vi "Module Top Level.vi"(8 "error in":errorcluster) -> (0 "error out":errorcluster)   [LabVIEW 2018, in "Fuel Farm.lvlib"]
doc: "This is the top level VI for this module. It uses a queue for communications and is stopped user a user event. The general architecture is similar to a simple queued message handler.\n\nThe VIs associated with this module are organized in a LabVIEW Library."
uses:
  Fuel Farm.lvlib
  Private Controls/UI 3 Data.ctl
  Top Level/Shared Controls/APU Setup File.ctl
  Testing UI 1/Private Controls/APU & ECU Controls.ctl
  Private Controls/Module Data.ctl
  Private Controls/Module Action.ctl
  Controller (Host)/Public Controls/APU Select.ctl
  <vilib>/event_ctls.llb/usereventprio.ctl
  Globals/Host Globals.vi
  Error Handler/Error Handler.lvlib
  Controller (Host)/Controller (Host).lvlib
  File IO/File IO.lvlib
  UDP Writer/PC UDP Writer.lvlib
  Testing UI 1/Testing UI 1.lvlib
panel:
  out "cRIO Status":bool
  in  "FuelSystem":bool caption="FUEL SYSTEM"
  in  "Pressure Regulator":dbl(slide)=4.0 min=4.0 max=20.0 step=0.1 scale=4.0..20.0 scale format="%_2g"
  out "01.00.9213.09":cluster{dbl, dbl, dbl, dbl}(slide)={0.0, 380.23952095808386, 305.38922155688624, 392.21556886227546} caption="Tamb" scale=0.0..200.0 scale format="%.2f F"
  out "01.00.9213.09":dbl(slide) caption="TFFT" scale=0.0..200.0
  out "C.36":dbl(slide) caption="Flow" scale=0.0..2000.0
  out "Fuel Pressure":dbl caption="PFI" format="%.2g"
  out "02.03.9227.03":dbl(slide)=100.0 caption="Level" scale=0.0..100.0
  out "UI 3 Data":T1
  out "STOP":bool
  # "Fuel Farm"
  # "Decrease"
  # "Increase"
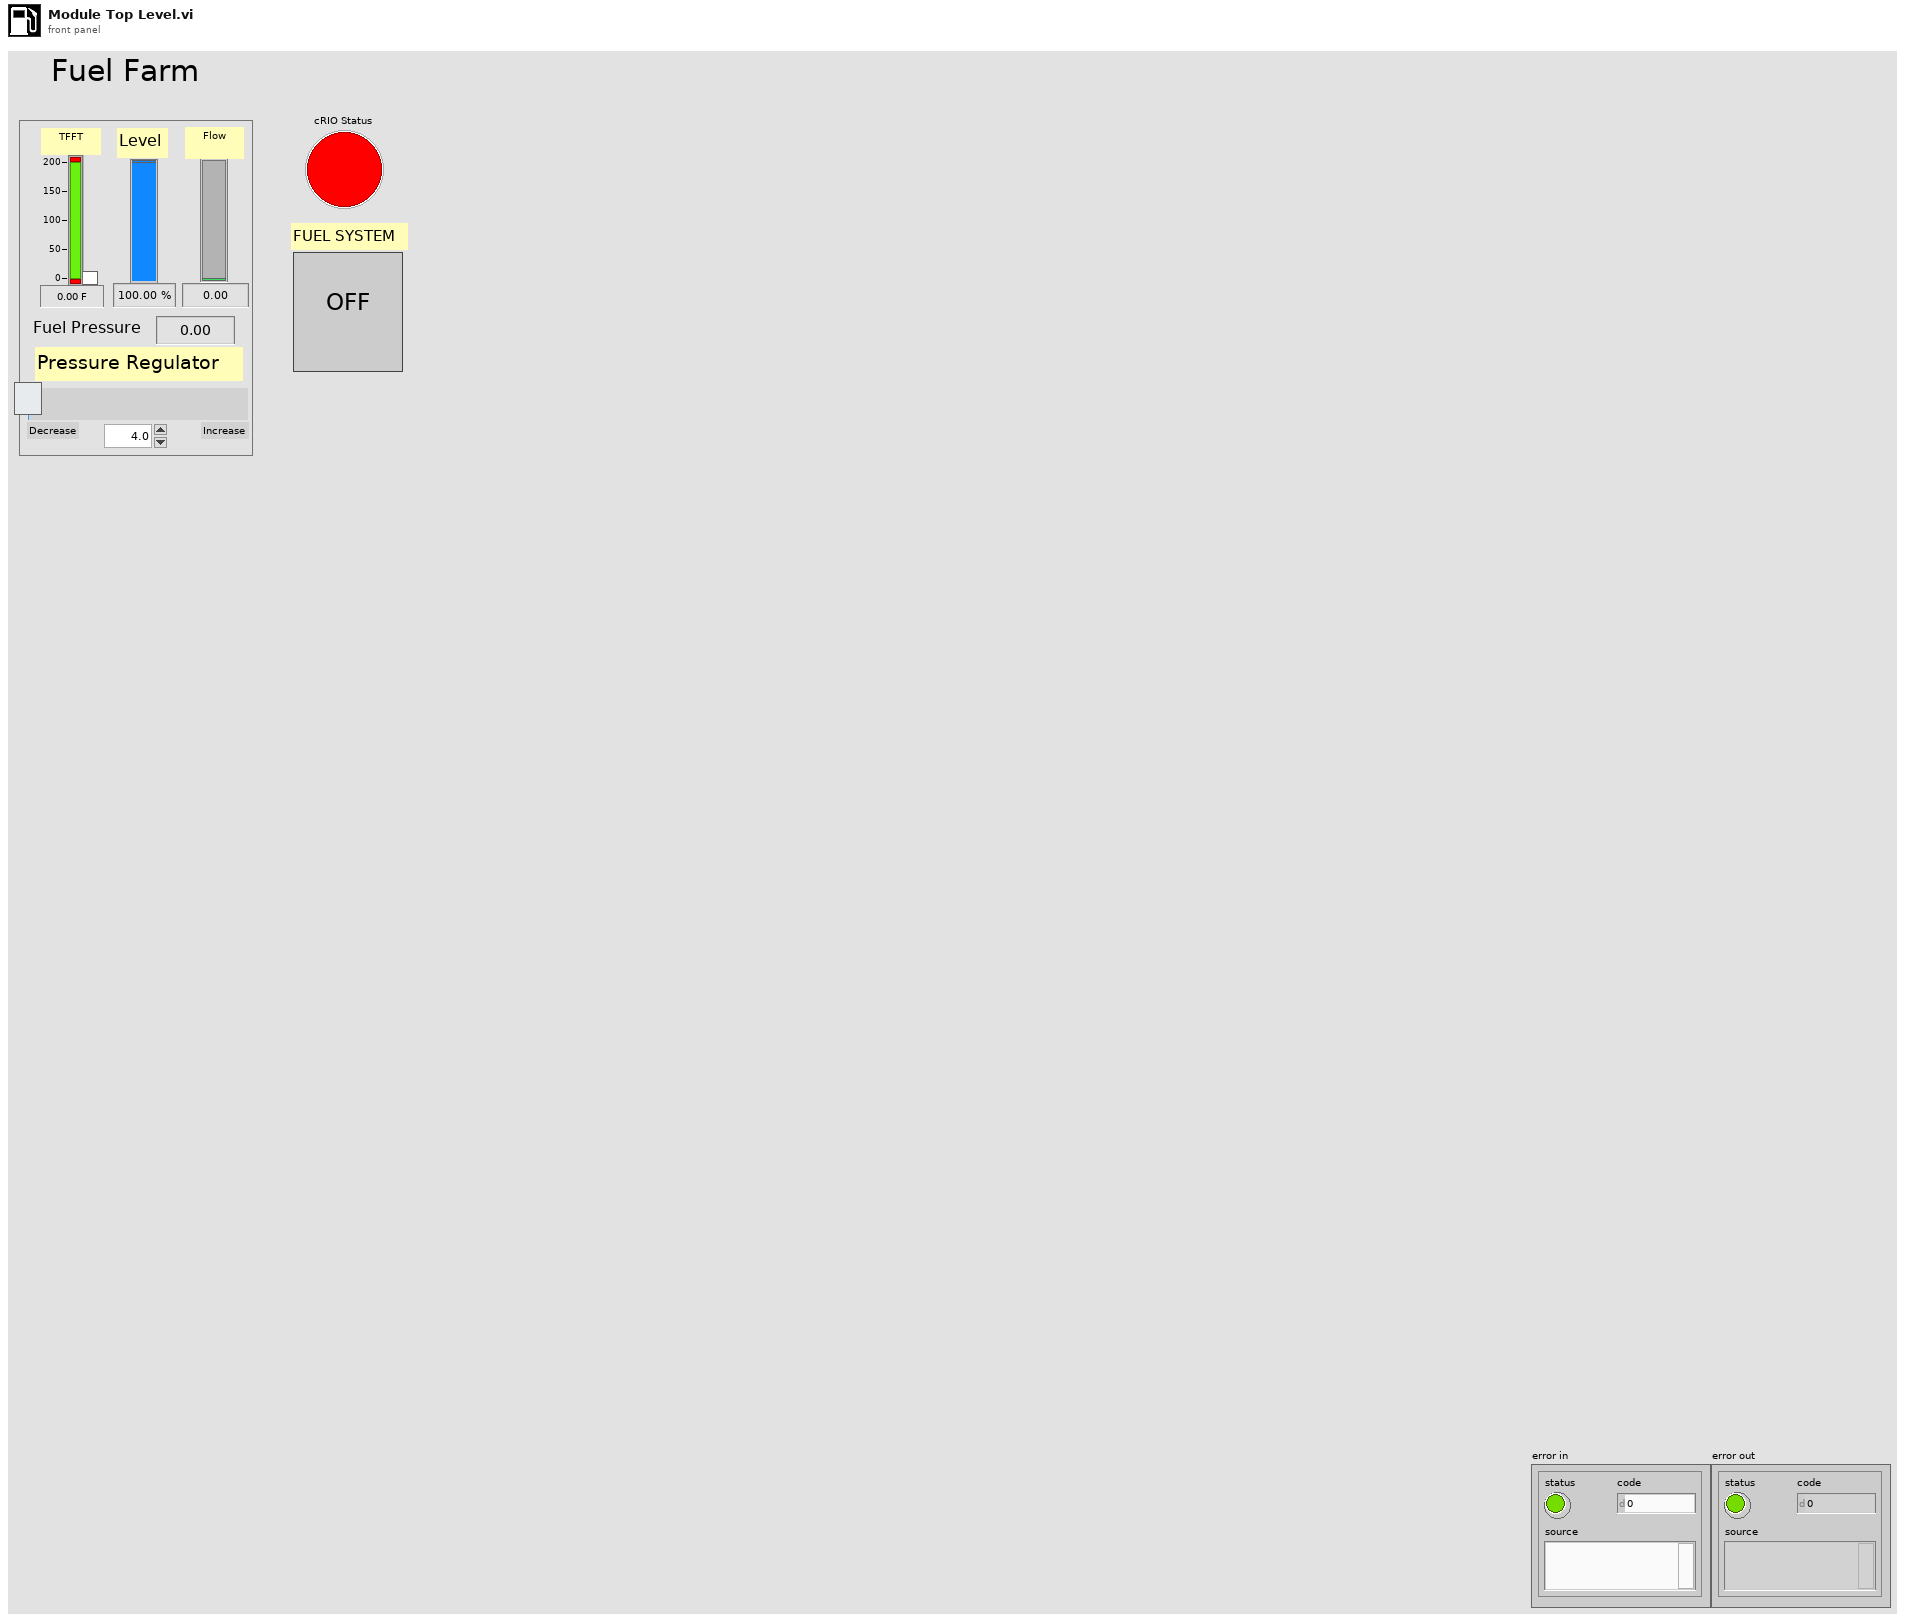
[diagram p1: front panel]
types:
  T1 = typedef "Fuel Farm.lvlib/UI 3 Data.ctl" = cluster{"APU Setup File":T2}
  T2 = typedef "APU Setup File.ctl" = cluster{"Sensor Info":string[][], "Variables":string[][], "CMM Table 106":string[][], "CMM Table 106B ":string[][], "Accel Config":string[][], "Report Sheet 1":string[][], "Report Sheet 2":string[][], "Report Sheet 3":string[][]}
  T3 = typedef "Testing UI 1.lvlib/APU & ECU Controls.ctl" = cluster{"02.01.9485.06":bool, "FuelPump":bool, "02.00.9485.01":bool, "02.00.9485.02":bool, "02.00.9485.03":bool, "02.00.9485.05":bool, "02.00.9485.04":bool, "02.00.9485.00":bool, "02.00.9485.07":bool, "02.01.9485.00":bool, "02.01.9485.01":bool}
  T4 = typedef "Controller (Host).lvlib/APU Select.ctl" = string
  T5 = enum32{"Invalid", "Standard", "Closed", "Hidden", "Minimized", "Maximized"}
  T6 = typedef "usereventprio.ctl" = enum32{"high priority", "normal priority"}
  T7 = typedef "Fuel Farm.lvlib/Module Data.ctl" = cluster{"Data":variant, "Action":T8}
  T8 = typedef "Fuel Farm.lvlib/Module Action.ctl" = enum8{"Init", "Open FP", "Timeout", "Error", "Exit"}
  T9 = typedef "Calculated Data.ctl" = cluster{"C.00":dbl, "C.01":dbl, "C.02":dbl, "C.03":dbl, "C.04":dbl, "C.05":dbl, "C.06":dbl, "C.07":dbl, "C.08":dbl, "C.09":dbl, "C.10":dbl, "C.11":dbl, "C.12":dbl, "C.13":dbl, "C.14":dbl, "C.15":dbl, "C.16":dbl, "C.17":dbl, "C.18":dbl, "C.19":dbl, "C.20":dbl, "C.21":dbl, "C.22":dbl, "C.23":dbl, "C.24":dbl, "C.25":dbl, "C.26":dbl, "C.27":dbl, "C.28":dbl, "C.29":dbl, "C.30":dbl, "C.31":dbl, "C.32":dbl, "C.33":dbl, "C.34":dbl, "C.35":dbl, "C.36":dbl, "C.37":dbl, "C.38":dbl, "C.39":dbl, "C.40":dbl, "C.41":dbl, "C.42":dbl, "C.43":dbl, "C.44":dbl, "C.45":dbl, "C.46":dbl, "C.47":dbl, "C.48":dbl, "C.49":dbl, "C.50":dbl, "C.51":dbl, "C.52":dbl, "C.53":dbl, "C.54":dbl, "C.55":dbl, "C.56":dbl, "C.57":dbl, "C.58":dbl, "C.59":dbl, "C.60":dbl, "C.61":dbl, "C.62":dbl}
  T10 = typedef "All Data Cluster.ctl" = cluster{"AI":T11, "Accel Data":cluster{"Accel RMS(in/sec2)":dbl[], "Accel Peak(in/sec2)":dbl[], "Velocity RMS(in/sec)":dbl[], "Velocity Peak(in/sec)":dbl[]}, "Temps":cluster{"01-00-9213":dbl[], "01-01-9213":dbl[], "01-02-9213":dbl[]}, "00-03-9402(RPM)":dbl[], "02-04-9871":dbl[], "ARINC":sgl[]}
  T11 = typedef "Acq Data.ctl" = cluster{"00-00-9220":dbl[], "00-01-9220":dbl[], "02-02-9219":dbl[], "02-03-9227":dbl[], "02-05-9205":dbl[]}
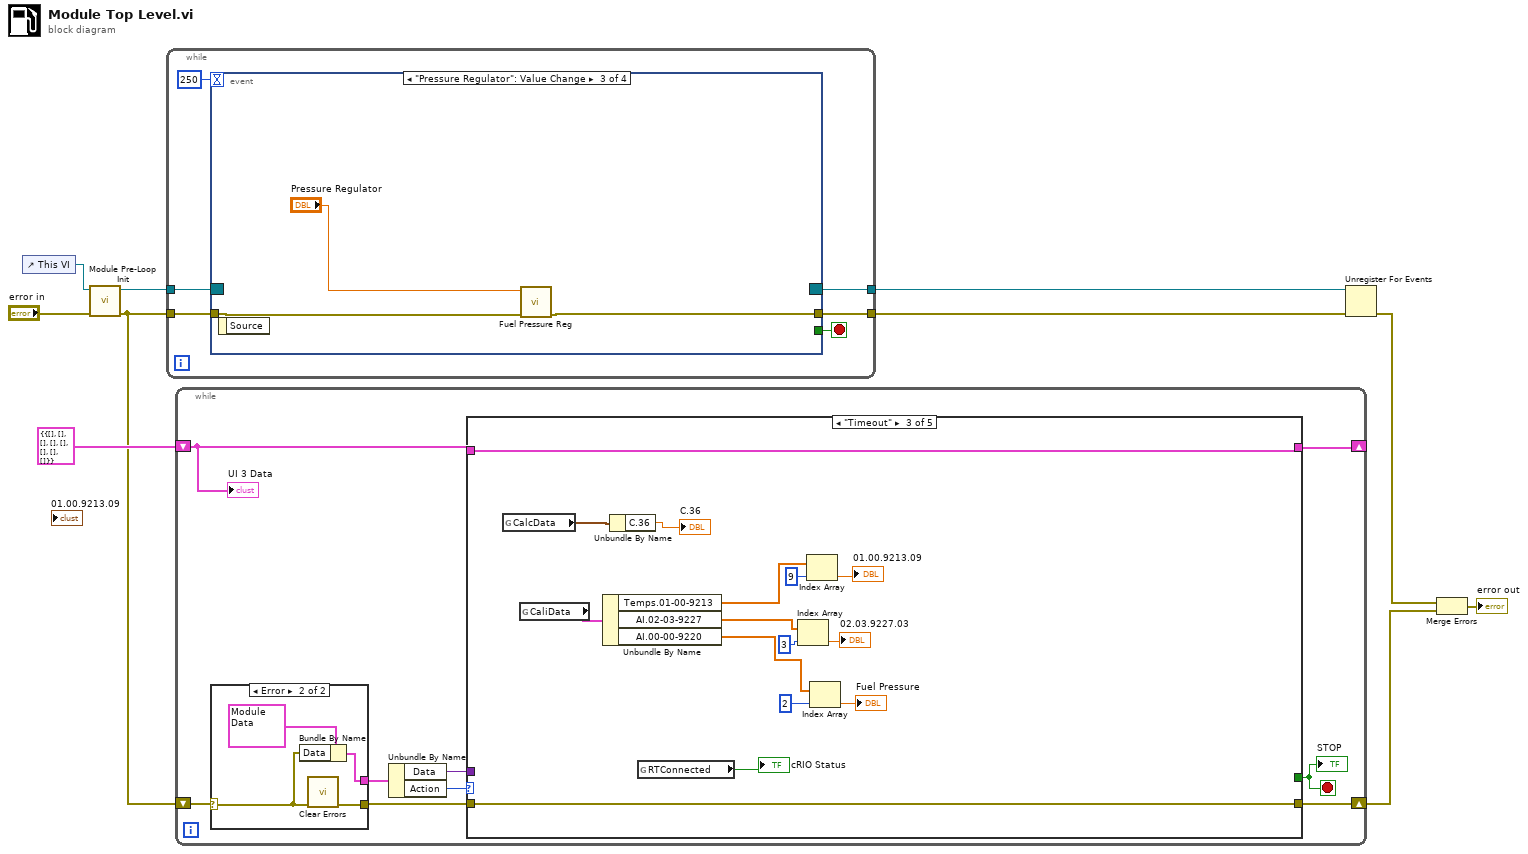
[diagram p0: block diagram]
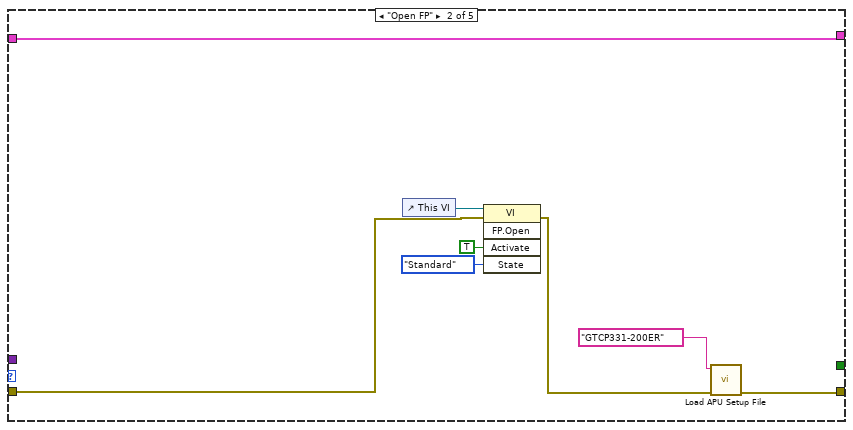
[diagram p3: hidden frame]
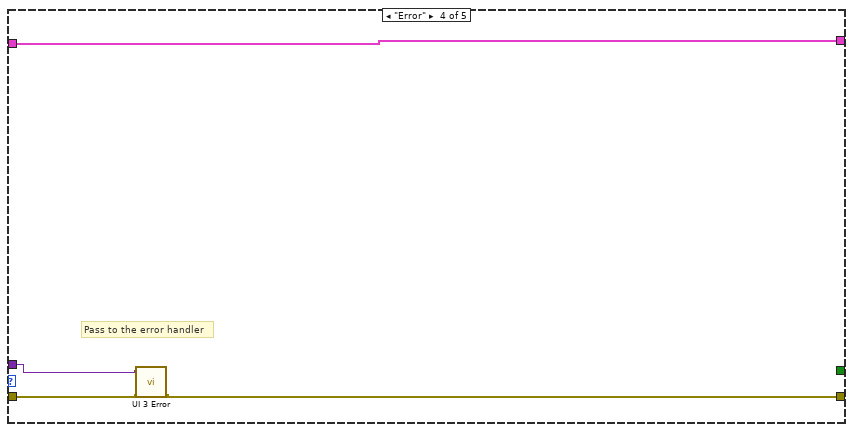
[diagram p4: hidden frame]
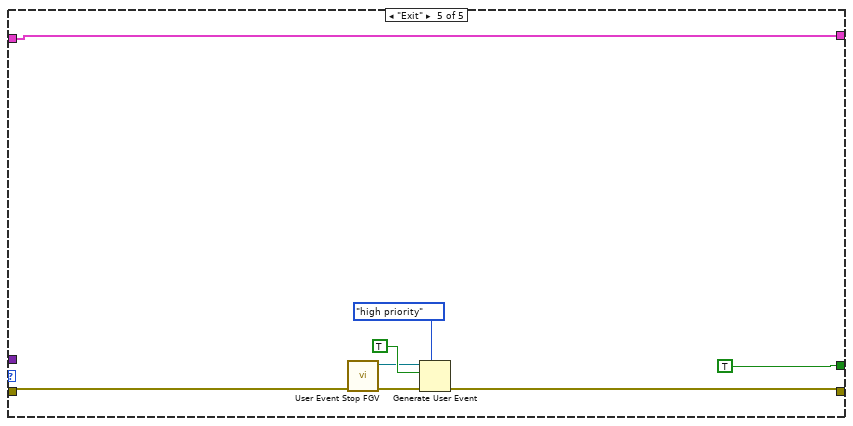
[diagram p5: hidden frame]
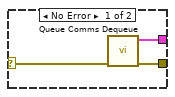
[diagram p6: hidden frame]
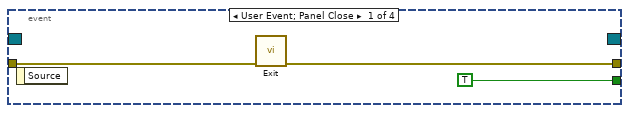
[diagram p7: hidden frame]
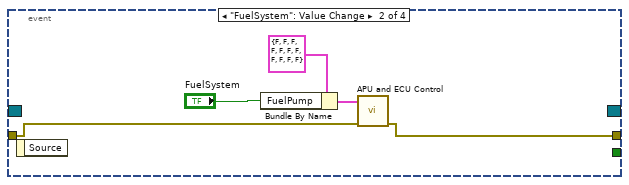
[diagram p8: hidden frame]
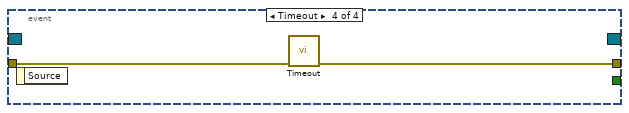
[diagram p9: hidden frame]
diagram:
  n1 = control-ref of="This VI"() -> (w10:refnum<vi>)
  n2 = call "Module Pre-Loop Init.vi"("error in (no error)"="error in", "Top Level VI Ref in"=w10) -> ("error out"=w1:errorcluster, "User Event Stop Ref"=w9:refnum<event-registration>)  [unwired: 8 in]
  n3 = while {
    tunnel: w9 -> [w16]
    tunnel: [w15] -> w7
    tunnel: w1 -> [w14]
    tunnel: [w12] -> w8
    stop <- w13 stop-if-true
    n4 = event shown="[2] \"Pressure Regulator\": Value Change" {
      selector: w16 -> [_ _ _ _]
      dyn-events: [_ _ _ _] -> w12
      timeout: 250 -> [_ _ _ _]
      tunnel: [w17 w21 w26 w28] -> w15
      tunnel: w14 -> [w18 w22 w27 w29]
      tunnel: [TRUE _ _ _] -> w13
      event User Event; Panel Close {
        n5 = event-data() -> ()  [unwired: 1 in, 1 out]
        n6 = call "Exit.vi"("error in"=w18) -> ("error out"=w17:errorcluster)  [unwired: 10 in]
      }
      event "FuelSystem": Value Change {
        n7 = event-data() -> ()  [unwired: 1 in, 1 out]
        n8 = Bundle By Name(cluster=T3 {"02.01.9485.06"=FALSE, "FuelPump"=FALSE, "02.00.9485.01"=FALSE, "02.00.9485.02"=FALSE, "02.00.9485.03"=FALSE, "02.00.9485.05"=FALSE, "02.00.9485.04"=FALSE, "02.00.9485.00"=FALSE, "02.00.9485.07"=FALSE, "02.01.9485.00"=FALSE, "02.01.9485.01"=FALSE} ("APU & ECU Control"), "FuelPump"="FuelSystem") -> (w24:T3)
        n9 = call "APU and ECU Control.vi"("error in (no error)"=w22, "APU & ECU Control"=w24) -> ("error out"=w21:errorcluster)  [unwired: 9 in]
      }
      event "Pressure Regulator": Value Change {
        n10 = event-data() -> ()  [unwired: 1 in, 1 out]
        n11 = call "Fuel Pressure Reg.vi"("error in (no error)"=w27, "Fuel Press Reg"="Pressure Regulator") -> ("error out"=w26:errorcluster)  [unwired: 9 in]
      }
      event Timeout {
        n12 = event-data() -> ()  [unwired: 1 in, 1 out]
        n13 = call "Timeout.vi"("error in (no error)"=w29) -> ("error out"=w28:errorcluster)  [unwired: 10 in]
      }
    }
  }
  n14 = while {
    shift-right: [w34] -> w6
    shift-left: w1 -> [w33]
    shift-right: [w31] -> _
    shift-left: T1 {"APU Setup File"={"Sensor Info"=[], "Variables"=[], "CMM Table 106"=[], "CMM Table 106B "=[], "Accel Config"=[], "Report Sheet 1"=[], "Report Sheet 2"=[], "Report Sheet 3"=[]}} -> [w32]
    stop <- w30 stop-if-true
    n15 = case shown="Error" w33 {
      selector: w33 -> [w77 w80]
      tunnel: [w78 w81] -> w38
      tunnel: [w76 w79] -> w35
      frame No Error {
        n16 = call "Queue Comms Dequeue.vi"("error in (no error)"=w77) -> ("error out"=w76:errorcluster, "element"=w78:T7)  [unwired: 9 in]
      }
      frame Error {
        n17 = Bundle By Name(cluster=T7 {"Data"=variant, "Action"=enum."Error"} ("element"), "Data"=w80) -> (w81:T7)
        n18 = call <vilib>:"Clear Errors.vi"("error in (no error)"=w80) -> ("error out"=w79:errorcluster)  [unwired: 5 in, 1 out]
      }
    }
    n19 = Unbundle By Name(w38) -> ("Data"=w36:variant, "Action"=w37:T8)
    n20 = case shown="\"Timeout\"" w37 {
      tunnel: w36 -> [_ _ _ w66 _]
      tunnel: w35 -> [w39 w44 w63 w65 w70]
      tunnel: [w39 w41 w63 w64 w68] -> w34
      tunnel: [_ _ _ _ TRUE] -> w30
      tunnel: w32 -> [w40 w48 w62 w67 w74]
      tunnel: [w40 w48 w62 w67 w74] -> w31
      frame "Init" {
      }
      frame "Open FP" {
        n21 = control-ref of="This VI"() -> (w47:refnum<vi>)
        n22 = invoke class="VI" method="FP.Open"(reference=w47, error in=w44, "Activate"=TRUE ("Activate?"), "State"=T5."Standard") -> (error out=w42:errorcluster)  [unwired: 1 in, 4 out]
        n23 = call "Load APU Setup File.vi"("error in (no error)"=w42, "APU Select"=T4 "GTCP331-200ER") -> ("error out"=w41:errorcluster)  [unwired: 9 in]
      }
      frame "Timeout" {
        n24 = global read "Host Globals.vi" "CalcData"() -> (w60:T9)
        n25 = global read "Host Globals.vi" "CaliData"() -> (w61:T10)
        n26 = Unbundle By Name(w61) -> ("Temps.01-00-9213"=w55:dbl[], "AI.02-03-9227"=w57:dbl[], "AI.00-00-9220"=w51:dbl[])
        n27 = Unbundle By Name(w60) -> ("C.36"=→"C.36":dbl)
        n28 = global read "Host Globals.vi" "RTConnected"() -> (→"cRIO Status":bool)
        n29 = Index Array(array=w57, index=3) -> (element=→"02.03.9227.03":dbl)
        n30 = Index Array(array=w55, index=9) -> (element=→"01.00.9213.09":dbl)
        n31 = Index Array(array=w51, index=2) -> (element=→"Fuel Pressure":dbl)
      }
      frame "Error" {
        # "Pass to the error handler"
        n32 = call "UI 3 Error.vi"("error in (no error)"=w65, "Data"=w66) -> ("error out"=w64:errorcluster)  [unwired: 9 in]
      }
      frame "Exit" {
        n33 = call "User Event Stop FGV.vi"("error in (no error)"=w70) -> ("error out"=w69:errorcluster, "User Event Stop"=w72:refnum<user-event>)  [unwired: 9 in]
        n34 = Generate User Event(priority (normal)=usereventprio."high priority", user event=w72, event data cluster=TRUE, error in=w69) -> (error out=w68:errorcluster)  [unwired: 1 out]
      }
    }
    "STOP" <- w30
    "UI 3 Data" <- w32
  }
  n35 = Unregister For Events(event registration refnum=w8, error in=w7) -> (error out=w4:errorcluster)
  n36 = Merge Errors(w4, w6) -> (→"error out":errorcluster)
